vi "sv_Flat Pink Noise Waveform.vi"(0 "noise density":dbl=0.1 format="%.2p", 1 "reset signal (F)":bool, 5 "lower cutoff freq":dbl=1.0 format="%#_2p", 9 "seed":i32=-1, 11 "error in (no error)":errorcluster, 12 "sampling info":cluster{"Fs":dbl, "#s":dbl}={"Fs"=1000.0, "#s"=1000.0} {"Fs" format="%.2p"}, 13 "reference freq (Hz)":dbl=1.0 format="%.2p") -> (4 "signal out":waveform(dbl), 6 "magnitude error (dB)":T2(graph), 8 "expected rms":dbl=1.0 format="%.2p", 10 "filter information":T1, 15 "error out":errorcluster)   [LabVIEW 2017]
uses:
  <vilib>/measure/NI_MABase.lvlib
  <vilib>/Analysis/NI_AALBase.lvlib
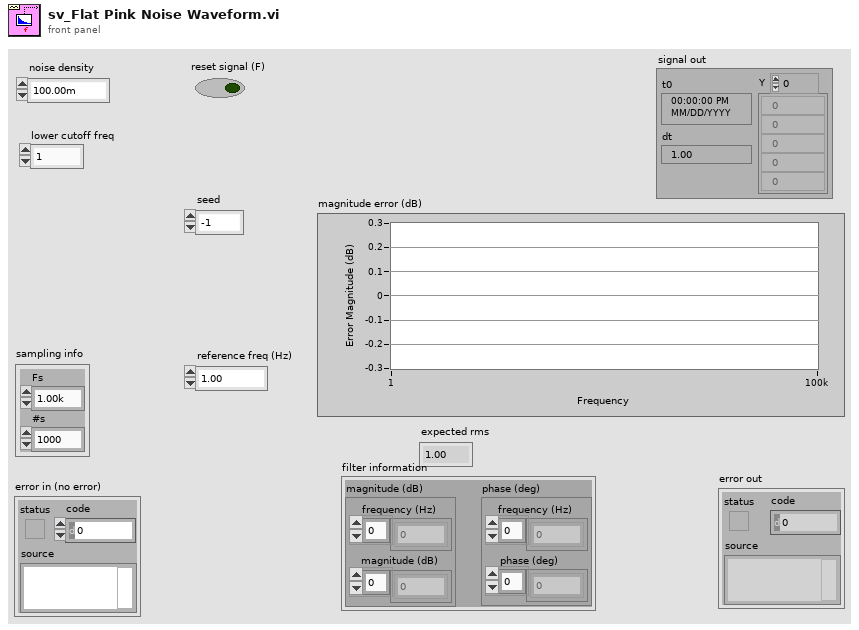
[diagram p1: front panel]
types:
  T1 = cluster{"magnitude (dB)":cluster{"frequency (Hz)":dbl[], "magnitude (dB)":dbl[]}, "phase (deg)":cluster{"frequency (Hz)":dbl[], "phase (deg)":dbl[]}}
  T2 = cluster{"frequency (Hz)":dbl[], "magnitude (dB)":dbl[]}
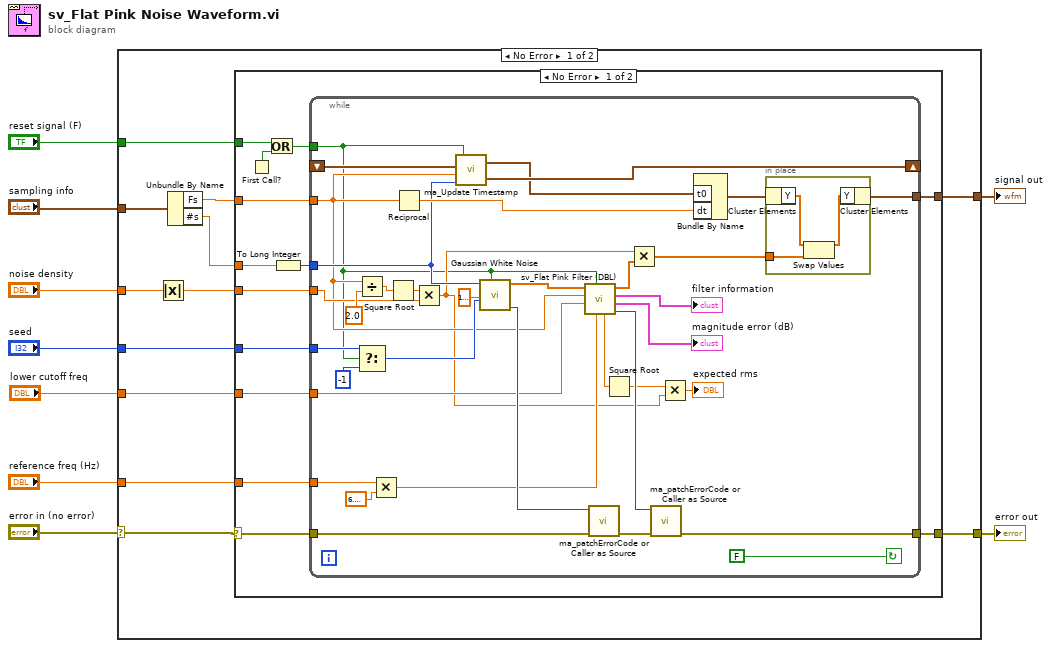
[diagram p0: block diagram]
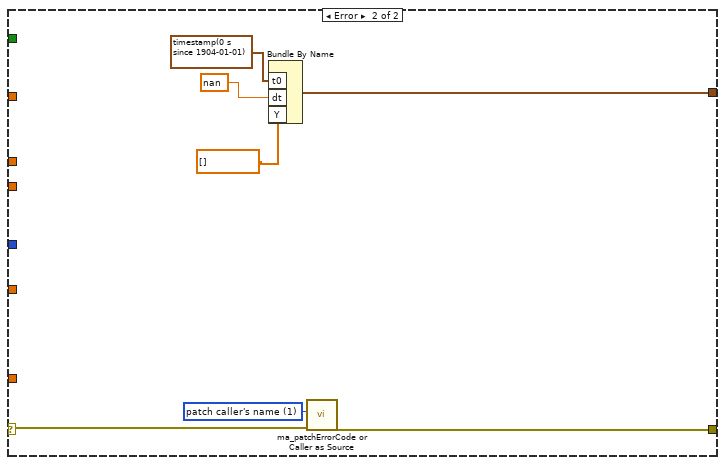
[diagram p2: hidden frame]
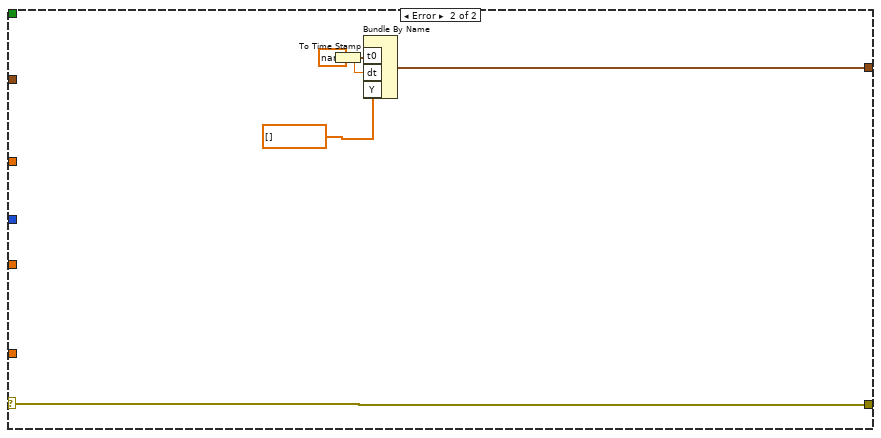
[diagram p3: hidden frame]
diagram:
  n1 = case shown="No Error" "error in (no error)" {
    selector: "error in (no error)" -> [w10 w85]
    tunnel: [w16 w85] -> w2
    tunnel: "sampling info" -> [w12 _]
    tunnel: [w19 w84] -> w4
    tunnel: "noise density" -> [w21 _]
    tunnel: "seed" -> [w20 _]
    tunnel: "lower cutoff freq" -> [w13 _]
    tunnel: "reference freq (Hz)" -> [w15 _]
    tunnel: "reset signal (F)" -> [w11 _]
    frame No Error {
      n2 = Absolute Value(x=w21) -> (abs(x)=w14:dbl)
      n3 = Unbundle By Name(w12) -> ("Fs"=w18:dbl, "#s"=w17:dbl)
      n4 = case shown="No Error" w10 {
        selector: w10 -> [w25 w74]
        tunnel: w14 -> [w34 _]
        tunnel: w20 -> [w33 _]
        tunnel: [w32 w78] -> w19
        tunnel: [w27 w76] -> w16
        tunnel: w18 -> [w31 _]
        tunnel: w17 -> [w30 _]
        tunnel: w13 -> [w28 _]
        tunnel: w15 -> [w26 _]
        tunnel: w11 -> [w22 _]
        frame No Error {
          n5 = First Call?() -> (First Call?: T/F=w24:bool)
          n6 = Or(x=w22, y=w24) -> (x .or. y?=w23:bool)
          n7 = To Long Integer(number=w30) -> (32bit integer=w29:i32)
          n8 = while {
            tunnel: w29 -> [w64]
            tunnel: w31 -> [w42]
            tunnel: [w37] -> w32
            shift-left: _ -> [w57]
            shift-right: [w59] -> _
            tunnel: w33 -> [w70]
            tunnel: w23 -> [w35]
            tunnel: w34 -> [w44]
            tunnel: w28 -> [w41]
            tunnel: [w63] -> w27
            tunnel: w25 -> [w60]
            tunnel: w26 -> [w50]
            stop <- FALSE continue-if-true
            n9 = Divide(x=w42, y=2.0) -> (x/y=w52:dbl)
            n10 = Select(t=w70, s=w35, f=-1) -> (s? t:f=w69:i32)
            n11 = Multiply(x=w50, y=6.283185307179586) -> (x*y=w48:dbl)
            n12 = Square Root(x=w52) -> (sqrt(x)=w53:dbl)
            n13 = Reciprocal(x=w42) -> (1/x=w68:dbl)
            n14 = Multiply(x=w53, y=w44) -> (x*y=w39:dbl)
            n15 = call <vilib>:"ma_Update Timestamp.vi"("samples"=w64, "Sampling Rate (Hz)"=w42, "tf previous"=w57, "Reset Generation"=w35) -> ("tf new"=w59:timestamp, "t0"=w58:timestamp)
            n16 = call <vilib>:"Gaussian White Noise.vi"("initialize?"=w35, "seed"=w69, "standard deviation"=1.0000000000000002, "samples"=w64) -> ("error"=w61:i32, "Gaussian noise pattern"=w65:dbl[])  [unwired: 6 in]
            n17 = call <vilib>:"sv_Flat Pink Filter (DBL).vi"("unity gain freq (rad/s)"=w48, "reset"=w35, "lower cutoff freq"=w41, "fs"=w42, "X"=w65) -> ("error"=w56:i32, "magnitude error (dB)"=→"magnitude error (dB)":T2, "filter information"=→"filter information":T1, "Filtered X"=w43:dbl[], "noise bandwidth"=w47:dbl)  [unwired: 2 in]
            n18 = call <vilib>:"ma_patchErrorCode or Caller as Source.vi"("error in (no error)"=w60, "error code"=w61) -> ("error out"=w62:errorcluster)  [unwired: 2 in, 7 out]
            n19 = Square Root(x=w47) -> (sqrt(x)=w46:dbl)
            n20 = Multiply(x=w39, y=w43) -> (x*y=w36:dbl[])
            n21 = call <vilib>:"ma_patchErrorCode or Caller as Source.vi"("error in (no error)"=w62, "error code"=w56) -> ("error out"=w63:errorcluster)  [unwired: 2 in, 7 out]
            n22 = Multiply(x=w46, y=w39) -> (x*y=→"expected rms":dbl)
            n23 = Bundle By Name("t0"=w58, "dt"=w68) -> (w38:waveform(dbl))  [unwired: 1 out]
            n24 = in-place {
              in-place-border: w36 -> [w72]
              n25 = in-place-cluster #1(w38) -> ("Y"=w71:dbl[])
              n26 = Swap Values(12:w71, 14:w72) -> (1:w73:dbl[])  [unwired: 1 in, 1 out]
              n27 = in-place-cluster #1("Y"=w73) -> (w37:waveform(dbl))
            }
          }
        }
        frame Error {
          w77 = u16 1 items=["patch error code", "patch caller's name"] ("operation")
          n28 = Bundle By Name("t0"=timestamp(0 s since 1904-01-01), "dt"=nan ("t0"), "Y"=dbl[] []) -> (w78:waveform(dbl))  [unwired: 1 out]
          n29 = call <vilib>:"ma_patchErrorCode or Caller as Source.vi"("error in (no error)"=w74, "operation"=w77) -> ("error out"=w76:errorcluster)  [unwired: 2 in, 7 out]
        }
      }
    }
    frame Error {
      w82 = nan ("t0")
      n30 = To Time Stamp(1:w82) -> (0:w81:timestamp)
      n31 = Bundle By Name("t0"=w81, "dt"=w82, "Y"=dbl[] []) -> (w84:waveform(dbl))  [unwired: 1 out]
    }
  }
  "error out" <- w2
  "signal out" <- w4
